vi "Read Module Menu Name.vi"(8 "error in":errorcluster, 11 "Profibus Module editor node in":refnum<class "Profibus Module editor node.lvclass">) -> (0 "error out":errorcluster, 2 "Menu Name":string, 3 "Profibus Module editor node out":refnum<class "Profibus Module editor node.lvclass">)   [LabVIEW 2013, in "Profibus Module editor node.lvclass"]
uses:
  Profibus Module editor node.lvclass
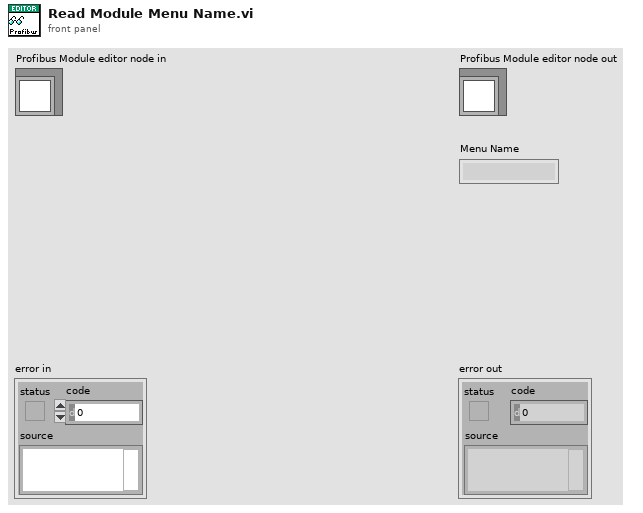
[diagram p1: front panel]
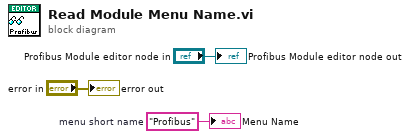
[diagram p0: block diagram]
diagram:
  w1 = "Profibus"  # menu short name
  "error out" <- "error in"
  "Profibus Module editor node out" <- "Profibus Module editor node in"
  "Menu Name" <- w1
